vi "VG_INIT.vi"() -> ()   [LabVIEW 2020]
panel:
  out "INIT?":dbl
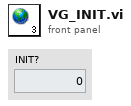
[diagram p1: front panel]
diagram:
